vi "loopdelay.vi"() -> ()   [LabVIEW 2011]
panel:
  out "Time array":u32[][](array[numeric])
  out "millisecond timer value":u32
  out "Loop Execution Time":u32
  out "Numeric":i32
  in  "milliseconds to wait":u32
  out "Array":i32[][](array[numeric])
  in  "Iterations":i32
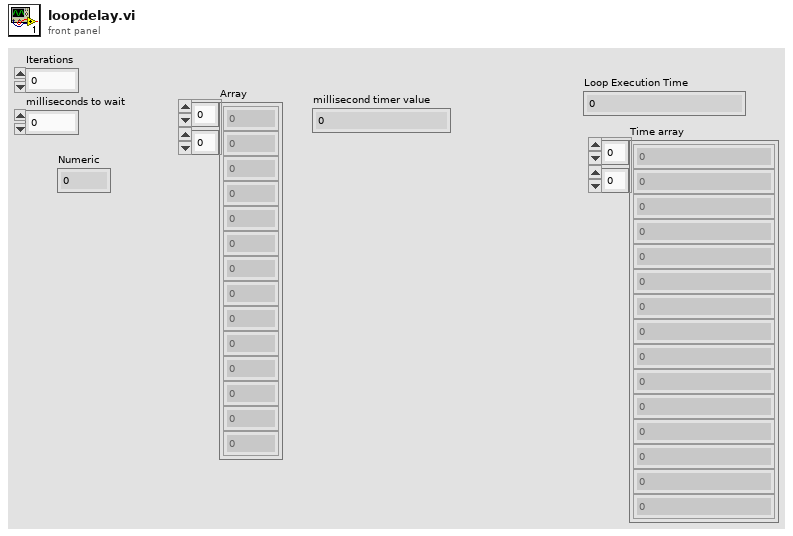
[diagram p1: front panel]
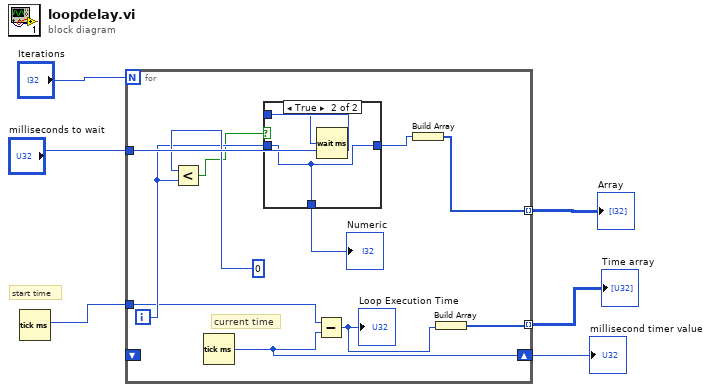
[diagram p0: block diagram]
diagram:
  # "start time"
  n1 = Tick Count (ms)() -> (millisecond timer value=w2:u32)
  n2 = for {
    N: "Iterations" -> [_]
    tunnel: [w15] -> w5 mode=indexing
    tunnel: "milliseconds to wait" -> [w17]
    shift-right: [w10] -> w3
    shift-left: _ -> [_]
    tunnel: w2 -> [w9]
    tunnel: [w7] -> w1 mode=indexing
    i -> [w12]
    # "current time"
    n3 = Less?(x=0, y=w12) -> (x < y?=w11:bool)
    n4 = Tick Count (ms)() -> (millisecond timer value=w10:u32)
    n5 = case shown="True" w11 {
      tunnel: w17 -> [_ w20]
      tunnel: [w18 w19] -> w16
      tunnel: w12 -> [w18 w19]
      tunnel: [w18 w19] -> w14
      frame False {
      }
      frame True {
        n6 = Wait (ms)(milliseconds to wait=w20) -> ()  [unwired: 1 out]
      }
    }
    "Numeric" <- w14
    n7 = Subtract(x=w9, y=w10) -> (x-y=w8:u32)
    "Loop Execution Time" <- w8
    n8 = Build Array(w16) -> (w15:i32[])
    n9 = Build Array(w8) -> (w7:u32[])
  }
  "Array" <- w5
  "millisecond timer value" <- w3
  "Time array" <- w1
